vi "Initialize Actor.vi"(7 "Host Name":string, 8 "error in (no error)":errorcluster, 9 "Actor Name":string, 10 "Message Broker Interface":refnum<class "Message Broker Interface.lvclass">, 11 "Mediated Synchronous Actor in":refnum<class "Mediated Synchronous Actor.lvclass">) -> (0 "error out":errorcluster, 3 "Mediated Synchronous Actor out":refnum<class "Mediated Synchronous Actor.lvclass">)   [LabVIEW 2016, in "Stream Mediator.lvlib" / "Mediated Synchronous Actor.lvclass"]
doc: "--\nCopyright © 2017 Composed SystemsI All rights reserved.\n\nAuthor: Jon McBee <jon.mcbee@composed.io>\n\nThis library is provided \"AS IS\" ,WITHOUT WARRANTIES OR\nCONDITIONS OF ANY KIND, either express or implied.\n\nComposed Systems -- composed.io\n\nStream 0.0.1.1\nJon McBee - Composed Systems\nCopyright (c) 2017, Composed Systems"
uses:
  <userlib>/Composed Systems/Stream/Mediator/Classes/Mediated Synchronous Actor/Mediated Synchronous Actor.lvclass
  C:/Program Files (x86)/National Instruments/LabVIEW 2016/user.lib/Composed Systems/Stream/Actor/Actor Class/Ancestral Actor.lvclass
  <userlib>/Composed Systems/Stream/Mediator/Classes/Message Broker Interface/Message Broker Interface.lvclass
  <userlib>/Composed Systems/Stream/Actor/Actor Class/Ancestral Actor.lvclass/Ancestral Actor.ctl
  <userlib>/Composed Systems/Stream/Mediator/Classes/Mediated Actor/Mediated Actor.lvclass
  <userlib>/Composed Systems/Stream/Actor/Actor Class/Ancestral Actor.lvclass
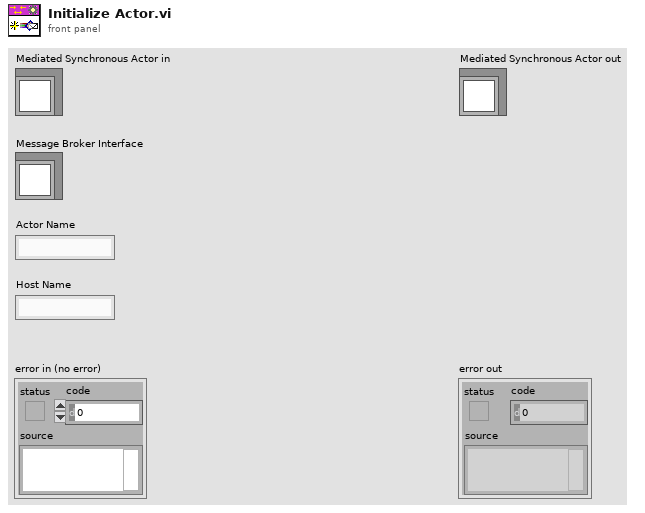
[diagram p1: front panel]
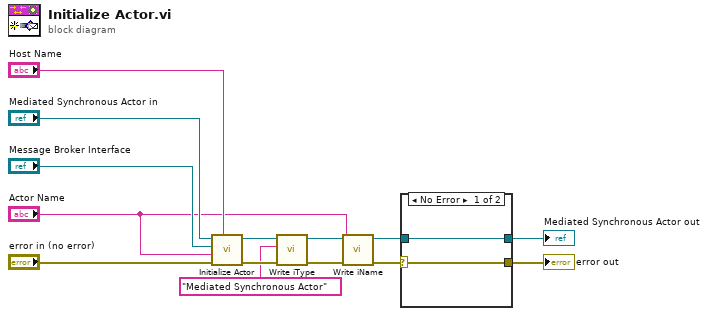
[diagram p0: block diagram]
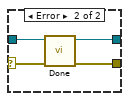
[diagram p2: hidden frame]
diagram:
  n1 = call-parent "Initialize Actor.vi"("Host Name"="Host Name", "error in (no error)"="error in (no error)", "Actor Name"="Actor Name", "Message Broker Interface"="Message Broker Interface", "Mediated Actor in"="Mediated Synchronous Actor in") -> ("error out"=w8:errorcluster, "Mediated Actor out"=w7:refnum<class "Mediated Synchronous Actor.lvclass">)  [unwired: 5 in]
  n2 = call <userlib>:"Write iType.vi"("error in (no error)"=w8, "iType"="Mediated Synchronous Actor", "Ancestral Actor in"=w7) -> ("error out"=w6:errorcluster, "Ancestral Actor out"=w4:refnum<class "Mediated Synchronous Actor.lvclass">)  [unwired: 7 in]
  n3 = call <userlib>:"Write iName.vi"("error in (no error)"=w6, "iName"="Actor Name", "Ancestral Actor in"=w4) -> ("error out"=w5:errorcluster, "Ancestral Actor out"=w3:refnum<class "Mediated Synchronous Actor.lvclass">)  [unwired: 7 in]
  n4 = case shown="No Error" w5 {
    selector: w5 -> [w15 w17]
    tunnel: [w15 w20] -> w10
    tunnel: w3 -> [w16 w19]
    tunnel: [w16 w18] -> w9
    frame No Error {
    }
    frame Error {
      n5 = call-dynamic "Done.vi"("error in (no error)"=w17, "Mediated Synchronous Actor in"=w19) -> ("error out"=w20:errorcluster, "Mediated Synchronous Actor out"=w18:refnum<class "Mediated Synchronous Actor.lvclass">)  [unwired: 8 in]
    }
  }
  "error out" <- w10
  "Mediated Synchronous Actor out" <- w9
